vi "Get Parent of Message.vi"(8 "error in":errorcluster, 11 "message":T1 format="%.0x") -> (0 "error out":errorcluster, 2 "parent of message":T1 format="%.0x", 3 "message out":T1 format="%.0x")   [LabVIEW 2023, in "Ballard MIL-STD-1553 Scripting.lvlib"]
uses:
  Ballard MIL-STD-1553 Scripting.lvlib
  <vilib>/NI VeriStand/Custom Device API/Custom Device Item Ref.ctl
  Constants.vi
  <vilib>/NI VeriStand/Custom Device API/Custom Device API.lvlib
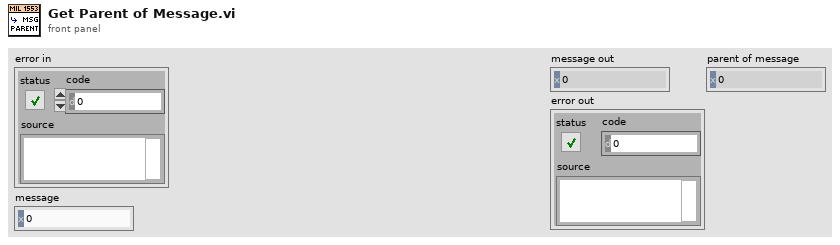
[diagram p1: front panel]
types:
  T1 = typedef "Custom Device API.lvlib/Custom Device Item Ref.ctl" = u64
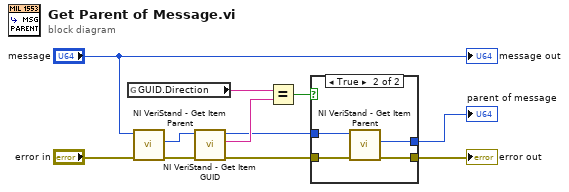
[diagram p0: block diagram]
diagram:
  n1 = global read "Constants.vi" "GUID.Direction"() -> (w1:string)
  n2 = call <vilib>:"NI VeriStand - Get Item Parent.vi"("error in (no error)"="error in", "Item Ref in"="message") -> ("error out"=w8:errorcluster, "Parent Ref"=w9:T1)  [unwired: 6 in, 2 out]
  n3 = call <vilib>:"NI VeriStand - Get Item GUID.vi"("error in (no error)"=w8, "Item Ref in"=w9) -> ("error out"=w4:errorcluster, "GUID"=w7:string, "Item Ref out"=w5:T1)  [unwired: 7 in]
  n4 = Equal?(x=w1, y=w7) -> (x = y?=w6:bool)
  n5 = case shown="True" w6 {
    tunnel: w5 -> [w12 w17]
    tunnel: w4 -> [w13 w16]
    tunnel: [w13 w15] -> w3
    tunnel: [w12 w14] -> w2
    frame False {
    }
    frame True {
      n6 = call <vilib>:"NI VeriStand - Get Item Parent.vi"("error in (no error)"=w16, "Item Ref in"=w17) -> ("error out"=w15:errorcluster, "Parent Ref"=w14:T1)  [unwired: 6 in, 2 out]
    }
  }
  "error out" <- w3
  "parent of message" <- w2
  "message out" <- "message"
